vi "Read Mathematics.vi"(8 "error in (no error)":errorcluster, 11 "VISA resource name":refnum<visa-resource-name>) -> (0 "error out":errorcluster, 2 "Processed data":dbl[](array[numeric]), 3 "VISA resource name out":refnum<visa-resource-name>)   [LabVIEW 2017, in "Sefram DAS220.lvlib"]
doc: "Read mathematical processes (up to 5).\nIf calculation is out of range or impossible, Nan is returned."
uses:
  <instrlib>/Sefram DAS220/Sefram DAS220.lvlib
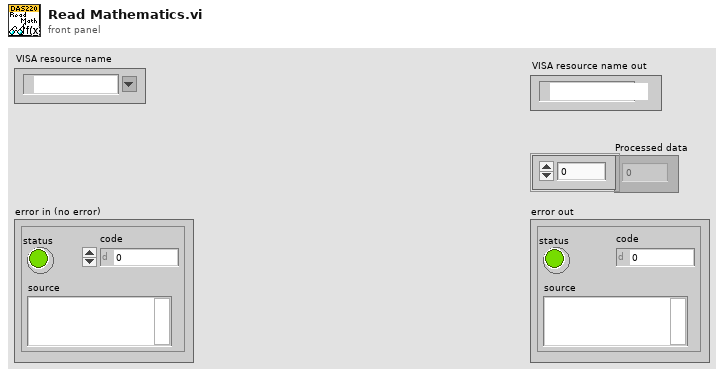
[diagram p1: front panel]
types:
  T1 = enum16{"big-endian, network order", "native, host order", "little-endian"}
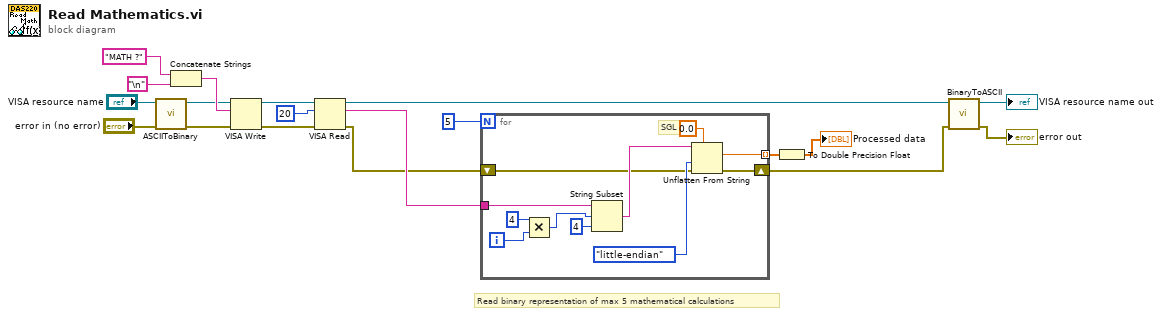
[diagram p0: block diagram]
diagram:
  # "Read binary representation of max 5 mathematical calculations"
  n1 = call <instrlib>:"ASCIIToBinary.vi"("error in (no error)"="error in (no error)", "VISA resource name"="VISA resource name") -> ("error out"=w7:errorcluster, "VISA resource name"=w8:refnum<visa-resource-name>)  [unwired: 8 in]
  n2 = Concatenate Strings("MATH ?" ("string"), "\n") -> (w17:string)
  n3 = VISA Write(VISA resource name=w8, write buffer=w17, error in (no error)=w7) -> (VISA resource name out=w15:refnum<visa-resource-name>, error out=w14:errorcluster)  [unwired: 1 out]
  n4 = VISA Read(VISA resource name=w15, byte count=u32 20, error in (no error)=w14) -> (VISA resource name out=w4:refnum<visa-resource-name>, read buffer=w11:string, error out=w10:errorcluster)  [unwired: 1 out]
  n5 = for {
    N: 5 -> [_]
    tunnel: [w21] -> w12 mode=indexing
    shift-right: [w22] -> w1
    shift-left: w10 -> [w23]
    tunnel: w11 -> [w20]
    i -> [w30]
    # "SGL"
    n6 = Multiply(x=4, y=w30) -> (x*y=w24:i32)
    n7 = String Subset(string=w20, offset (0)=w24, length (rest)=4 ("length (rest)")) -> (substring=w28:string)
    n8 = Unflatten From String(type=sgl 0.0, binary string=w28, byte order (0:big-endian, network order)=T1."little-endian", error in (no error)=w23) -> (value=w21:sgl, error out=w22:errorcluster)  [unwired: 1 in, 1 out]
  }
  n9 = To Double Precision Float(number=w12) -> (double precision float=→"Processed data":dbl[])
  n10 = call <instrlib>:"BinaryToASCII.vi"("error in (no error)"=w1, "VISA resource name"=w4) -> ("error out"=→"error out":errorcluster, "VISA resource name"=→"VISA resource name out":refnum<visa-resource-name>)  [unwired: 8 in]
